vi "PLE_launcher.vi"() -> ()   [LabVIEW 2023]
uses:
  UIs/SpectrometerUI/SpectrometerUI/SpectrometerUI.lvclass
  <vilib>/ActorFramework/Actor/Actor.lvclass
panel:
  in  "Stop":bool
  in  "PLE Scan UI":bool
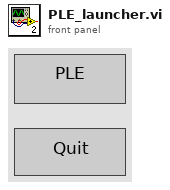
[diagram p1: front panel]
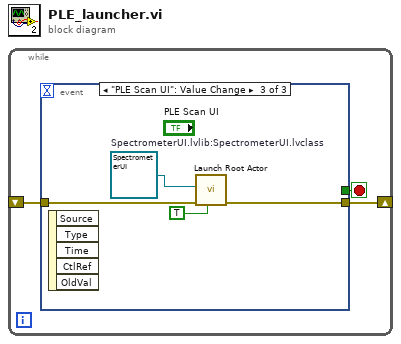
[diagram p0: block diagram]
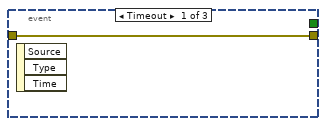
[diagram p2: hidden frame]
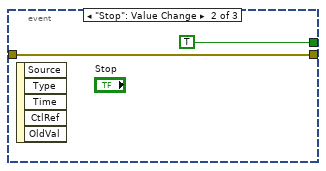
[diagram p3: hidden frame]
diagram:
  n1 = while {
    shift-right: [w2] -> _
    shift-left: _ -> [w1]
    stop <- w3 stop-if-true
    n2 = event shown="[2] \"PLE Scan UI\": Value Change" {
      selector: _ -> [_ _ _]
      dyn-events: _ -> [_ _ _]
      timeout: _ -> [_ _ _]
      tunnel: [_ TRUE _] -> w3
      tunnel: [w4 w5 w9] -> w2
      tunnel: w1 -> [w4 w5 w8]
      event Timeout {
        n3 = event-data() -> ()  [unwired: 1 in, 3 out]
      }
      event "Stop": Value Change {
        n4 = event-data() -> ()  [unwired: 1 in, 5 out]
      }
      event "PLE Scan UI": Value Change {
        w7 = refnum<class "SpectrometerUI.lvclass"> refnum  # SpectrometerUI.lvlib:SpectrometerUI.lvclass
        n5 = event-data() -> ()  [unwired: 1 in, 5 out]
        n6 = call <vilib>:"Launch Root Actor.vi"("Open Actor Core front panel? (F)"=TRUE, "error in (no error)"=w8, "Actor"=w7) -> ("error out"=w9:errorcluster)  [unwired: 7 in, 1 out]
      }
    }
  }
